vi "Set wavegen PULSe signal parameters.vi"(7 "Pulse Width (s)":dbl, 8 "error in (no error)":errorcluster {"code" format="%.0x"}, 9 "Wavegen parameters in":T2={"Frequency (Hz)"=1000.0, "Amplitude (V)"=1.0, "Offset (V)"=0.0, "Load Impedance"=enum."ONEMeg"} {"Offset (V)" format="%#_13g"; "Amplitude (V)" format="%#_13g"; "Frequency (Hz)" min=0.1 max=20000000.0 format="%#_13g"}, 11 "instrument handle in":refnum<k15>) -> (0 "error out":errorcluster, 2 "log string out":string, 3 "instrument handle out":refnum<k15>)   [LabVIEW 2017]
uses:
  Load Impedance.ctl
  Waveform type.ctl
  <instrlib>/Keysight InfiniiVision/Keysight InfiniiVision.lvlib
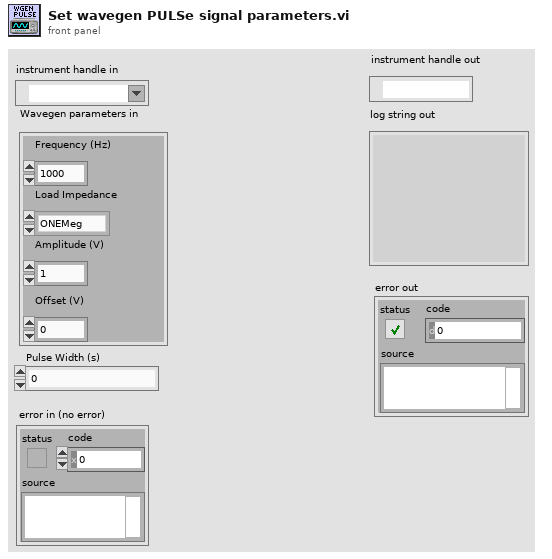
[diagram p1: front panel]
types:
  T1 = typedef "Load Impedance.ctl" = enum16{"ONEMeg", "FIFTy"}
  T2 = cluster{"Frequency (Hz)":dbl, "Amplitude (V)":dbl, "Offset (V)":dbl, "Load Impedance":T1}
  T3 = typedef "Waveform type.ctl" = enum16{"SINe", "SQUare", "RAMP", "PULSe", "DC", "NOISe"}
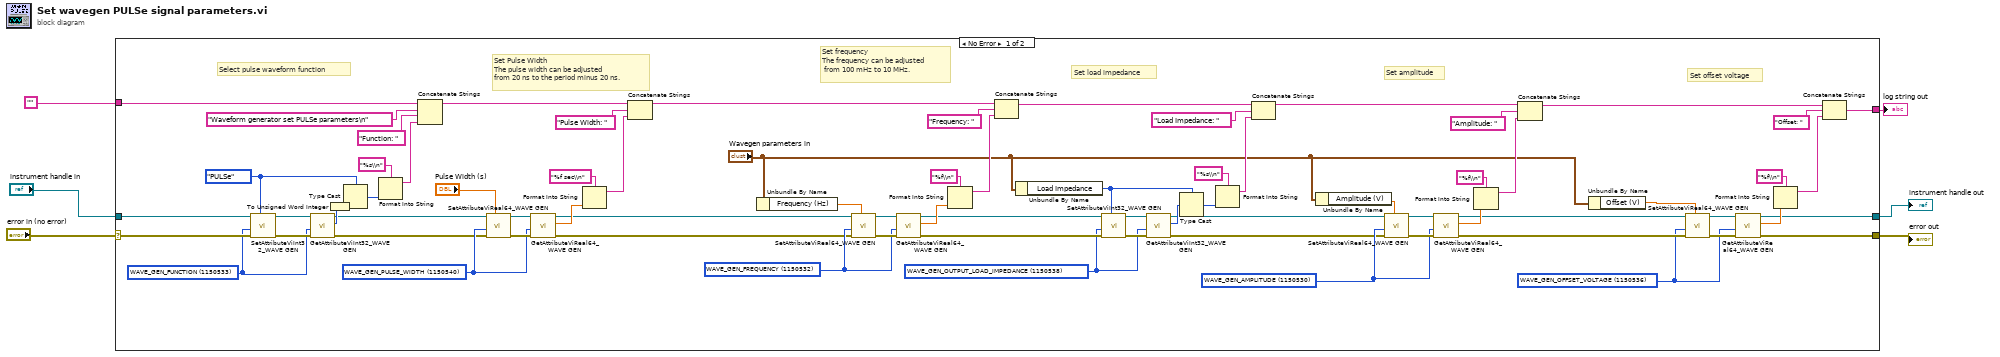
[diagram p0: block diagram]
diagram:
  n1 = case shown="No Error" "error in (no error)" {
    selector: "error in (no error)" -> [w79 w81]
    tunnel: "instrument handle in" -> [w80 w82]
    tunnel: [w48 w82] -> w2
    tunnel: [w47 w81] -> w1
    tunnel: [w46 w83] -> w3
    tunnel: "" ("log string in") -> [w44 w83]
    frame No Error {
      w13 = u32 1150540 items=["FM_DEVIATION"=1150548, "FM_FREQUENCY"=1150549, "FSK_FREQUENCY"=1150550, "FSK_MODULATION_RATE"=1150551, "MODULATION_RAMP_SYMMETRY"=1150553, "WAVE_GEN_AM_DEPTH"=1150546, "WAVE_GEN_AM_FREQUENCY"=1150547, "WAVE_GEN_AMPLITUDE"=1150530, "WAVE_GEN_DUTY_CYCLE"=1150531, "WAVE_GEN_FREQUENCY"=1150532, "WAVE_GEN_HIGH_VOLTAGE"=1150534, "WAVE_GEN_LOW_VOLTAGE"=1150535, "WAVE_GEN_OFFSET_VOLTAGE"=1150536, "WAVE_GEN_PERIOD"=1150539, "WAVE_GEN_PULSE_WIDTH"=1150540, "WAVE_GEN_RAMP_SYMMETRY"=1150541] ("AttributeID")
      w36 = u32 1150538 items=["ARBITRARY_BYTE_ORDER"=1150415, "MODULATION_FUNCTION"=1150552, "MODULATION_TYPE"=1150555, "TRACKING_PHASE"=1150659, "WAVE_GEN_ADDITIONAL_NOISE"=1150529, "WAVE_GEN_ARBITRARY_BYTE_ORDER"=1150544, "WAVE_GEN_FUNCTION"=1150533, "WAVE_GEN_OUTPUT_LOAD_IMPEDANCE"=1150538, "WAVE_GEN_OUTPUT_MODE"=1150658] ("AttributeID")
      w41 = u32 1150536 items=["FM_DEVIATION"=1150548, "FM_FREQUENCY"=1150549, "FSK_FREQUENCY"=1150550, "FSK_MODULATION_RATE"=1150551, "MODULATION_RAMP_SYMMETRY"=1150553, "WAVE_GEN_AM_DEPTH"=1150546, "WAVE_GEN_AM_FREQUENCY"=1150547, "WAVE_GEN_AMPLITUDE"=1150530, "WAVE_GEN_DUTY_CYCLE"=1150531, "WAVE_GEN_FREQUENCY"=1150532, "WAVE_GEN_HIGH_VOLTAGE"=1150534, "WAVE_GEN_LOW_VOLTAGE"=1150535, "WAVE_GEN_OFFSET_VOLTAGE"=1150536, "WAVE_GEN_PERIOD"=1150539, "WAVE_GEN_PULSE_WIDTH"=1150540, "WAVE_GEN_RAMP_SYMMETRY"=1150541] ("AttributeID")
      w70 = Waveform_type."PULSe"
      w42 = u32 1150530 items=["FM_DEVIATION"=1150548, "FM_FREQUENCY"=1150549, "FSK_FREQUENCY"=1150550, "FSK_MODULATION_RATE"=1150551, "MODULATION_RAMP_SYMMETRY"=1150553, "WAVE_GEN_AM_DEPTH"=1150546, "WAVE_GEN_AM_FREQUENCY"=1150547, "WAVE_GEN_AMPLITUDE"=1150530, "WAVE_GEN_DUTY_CYCLE"=1150531, "WAVE_GEN_FREQUENCY"=1150532, "WAVE_GEN_HIGH_VOLTAGE"=1150534, "WAVE_GEN_LOW_VOLTAGE"=1150535, "WAVE_GEN_OFFSET_VOLTAGE"=1150536, "WAVE_GEN_PERIOD"=1150539, "WAVE_GEN_PULSE_WIDTH"=1150540, "WAVE_GEN_RAMP_SYMMETRY"=1150541] ("AttributeID")
      w43 = u32 1150532 items=["FM_DEVIATION"=1150548, "FM_FREQUENCY"=1150549, "FSK_FREQUENCY"=1150550, "FSK_MODULATION_RATE"=1150551, "MODULATION_RAMP_SYMMETRY"=1150553, "WAVE_GEN_AM_DEPTH"=1150546, "WAVE_GEN_AM_FREQUENCY"=1150547, "WAVE_GEN_AMPLITUDE"=1150530, "WAVE_GEN_DUTY_CYCLE"=1150531, "WAVE_GEN_FREQUENCY"=1150532, "WAVE_GEN_HIGH_VOLTAGE"=1150534, "WAVE_GEN_LOW_VOLTAGE"=1150535, "WAVE_GEN_OFFSET_VOLTAGE"=1150536, "WAVE_GEN_PERIOD"=1150539, "WAVE_GEN_PULSE_WIDTH"=1150540, "WAVE_GEN_RAMP_SYMMETRY"=1150541] ("AttributeID")
      w76 = u32 1150533 items=["ARBITRARY_BYTE_ORDER"=1150415, "MODULATION_FUNCTION"=1150552, "MODULATION_TYPE"=1150555, "TRACKING_PHASE"=1150659, "WAVE_GEN_ADDITIONAL_NOISE"=1150529, "WAVE_GEN_ARBITRARY_BYTE_ORDER"=1150544, "WAVE_GEN_FUNCTION"=1150533, "WAVE_GEN_OUTPUT_LOAD_IMPEDANCE"=1150538, "WAVE_GEN_OUTPUT_MODE"=1150658] ("AttributeID")
      # "Set Pulse Width\nThe pulse width can be adjusted \nfrom 20 ns to the period minus 20 ns."
      # "Set load impedance"
      # "Set offset voltage"
      # "Set amplitude"
      # "Set frequency\nThe frequency can be adjusted\n from 100 mHz to 10 MHz."
      # "Select pulse waveform function"
      n2 = call <instrlib>:"SetAttributeViInt32_WAVE GEN.vi"("AttributeValue"=w70, "error in (no error)"=w79, "AttributeID"=w76, "instrument handle"=w80) -> ("error out"=w77:errorcluster, "instrument handle out"=w78:refnum<k15>)  [unwired: 6 in]
      n3 = call <instrlib>:"GetAttributeViInt32_WAVE GEN.vi"("error in (no error)"=w77, "AttributeID"=w76, "instrument handle"=w78) -> ("error out"=w10:errorcluster, "AttributeValue"=w71:i32, "instrument handle out"=w11:refnum<k15>)  [unwired: 6 in]
      n4 = To Unsigned Word Integer(number=w71) -> (unsigned 16bit integer=w7:u16)
      n5 = Type Cast(type=w70, x=w7) -> (*(type *) &x=w69:T3)
      n6 = Format Into String(format string="%s\\n", w69) -> (resulting string=w68:string)  [unwired: 2 in, 1 out]
      n7 = Concatenate Strings(w44, "Waveform generator set PULSe parameters\n" ("string"), "Function: " ("string"), w68) -> (w15:string)
      n8 = call <instrlib>:"SetAttributeViReal64_WAVE GEN.vi"("AttributeValue"="Pulse Width (s)", "error in (no error)"=w10, "AttributeID"=w13, "instrument handle"=w11) -> ("error out"=w20:errorcluster, "instrument handle out"=w21:refnum<k15>)  [unwired: 6 in]
      n9 = call <instrlib>:"GetAttributeViReal64_WAVE GEN.vi"("error in (no error)"=w20, "AttributeID"=w13, "instrument handle"=w21) -> ("error out"=w8:errorcluster, "AttributeValue"=w19:dbl, "instrument handle out"=w9:refnum<k15>)  [unwired: 6 in]
      n10 = Format Into String(format string="%f sec\\n", w19) -> (resulting string=w16:string)  [unwired: 2 in, 1 out]
      n11 = Concatenate Strings(w15, "Pulse Width: " ("string"), w16) -> (w14:string)
      n12 = Unbundle By Name("Wavegen parameters in") -> ("Frequency (Hz)"=w26:dbl)
      n13 = call <instrlib>:"SetAttributeViReal64_WAVE GEN.vi"("AttributeValue"=w26, "error in (no error)"=w8, "AttributeID"=w43, "instrument handle"=w9) -> ("error out"=w74:errorcluster, "instrument handle out"=w75:refnum<k15>)  [unwired: 6 in]
      n14 = call <instrlib>:"GetAttributeViReal64_WAVE GEN.vi"("error in (no error)"=w74, "AttributeID"=w43, "instrument handle"=w75) -> ("error out"=w37:errorcluster, "AttributeValue"=w67:dbl, "instrument handle out"=w38:refnum<k15>)  [unwired: 6 in]
      n15 = Format Into String(format string="%f\\n", w67) -> (resulting string=w63:string)  [unwired: 2 in, 1 out]
      n16 = Concatenate Strings(w14, "Frequency: " ("string"), w63) -> (w31:string)
      n17 = Unbundle By Name("Wavegen parameters in") -> ("Load Impedance"=w25:T1)
      n18 = call <instrlib>:"SetAttributeViInt32_WAVE GEN.vi"("AttributeValue"=w25, "error in (no error)"=w37, "AttributeID"=w36, "instrument handle"=w38) -> ("error out"=w40:errorcluster, "instrument handle out"=w39:refnum<k15>)  [unwired: 6 in]
      n19 = call <instrlib>:"GetAttributeViInt32_WAVE GEN.vi"("error in (no error)"=w40, "AttributeID"=w36, "instrument handle"=w39) -> ("error out"=w28:errorcluster, "AttributeValue"=w33:i32, "instrument handle out"=w27:refnum<k15>)  [unwired: 6 in]
      n20 = Type Cast(type=w25, x=w33) -> (*(type *) &x=w35:T1)
      n21 = Format Into String(format string="%s\\n", w35) -> (resulting string=w30:string)  [unwired: 2 in, 1 out]
      n22 = Concatenate Strings(w31, "Load Impedance: " ("string"), w30) -> (w29:string)
      n23 = Unbundle By Name("Wavegen parameters in") -> ("Amplitude (V)"=w24:dbl)
      n24 = call <instrlib>:"SetAttributeViReal64_WAVE GEN.vi"("AttributeValue"=w24, "error in (no error)"=w28, "AttributeID"=w42, "instrument handle"=w27) -> ("error out"=w72:errorcluster, "instrument handle out"=w73:refnum<k15>)  [unwired: 6 in]
      n25 = call <instrlib>:"GetAttributeViReal64_WAVE GEN.vi"("error in (no error)"=w72, "AttributeID"=w42, "instrument handle"=w73) -> ("error out"=w51:errorcluster, "AttributeValue"=w53:dbl, "instrument handle out"=w52:refnum<k15>)  [unwired: 6 in]
      n26 = Format Into String(format string="%f\\n", w53) -> (resulting string=w59:string)  [unwired: 2 in, 1 out]
      n27 = Concatenate Strings(w29, "Amplitude: " ("string"), w59) -> (w49:string)
      n28 = Unbundle By Name("Wavegen parameters in") -> ("Offset (V)"=w23:dbl)
      n29 = call <instrlib>:"SetAttributeViReal64_WAVE GEN.vi"("AttributeValue"=w23, "error in (no error)"=w51, "AttributeID"=w41, "instrument handle"=w52) -> ("error out"=w57:errorcluster, "instrument handle out"=w58:refnum<k15>)  [unwired: 6 in]
      n30 = call <instrlib>:"GetAttributeViReal64_WAVE GEN.vi"("error in (no error)"=w57, "AttributeID"=w41, "instrument handle"=w58) -> ("error out"=w47:errorcluster, "AttributeValue"=w50:dbl, "instrument handle out"=w48:refnum<k15>)  [unwired: 6 in]
      n31 = Format Into String(format string="%f\\n", w50) -> (resulting string=w54:string)  [unwired: 2 in, 1 out]
      n32 = Concatenate Strings(w49, "Offset: " ("string"), w54) -> (w46:string)
    }
    frame Error {
    }
  }
  "log string out" <- w3
  "instrument handle out" <- w2
  "error out" <- w1
